vi "PNG Read.vi"(8 "error in (no error)":errorcluster, 11 "Image Path (*.png)":path) -> (0 "error out":errorcluster, 2 "Chunks":T1[](array[typedef]) {"CRC" format="%08x"}, 3 "dup Image Path":path)   [LabVIEW 2018, in "Export-Built-ins.lvlib"]
doc: "Returns the PNG image chunks from the <b>Image Path (*.png)</b>.\n\n<b>Errors:</b>\n1059: \"Unsupported file type\" if <b>Image Path (*.png)</b> is not a valid PNG file.\n\nCreated by: Ryan Pacini"
uses:
  Export-Built-ins.lvlib
  Controls/PNG Chunk.ctl
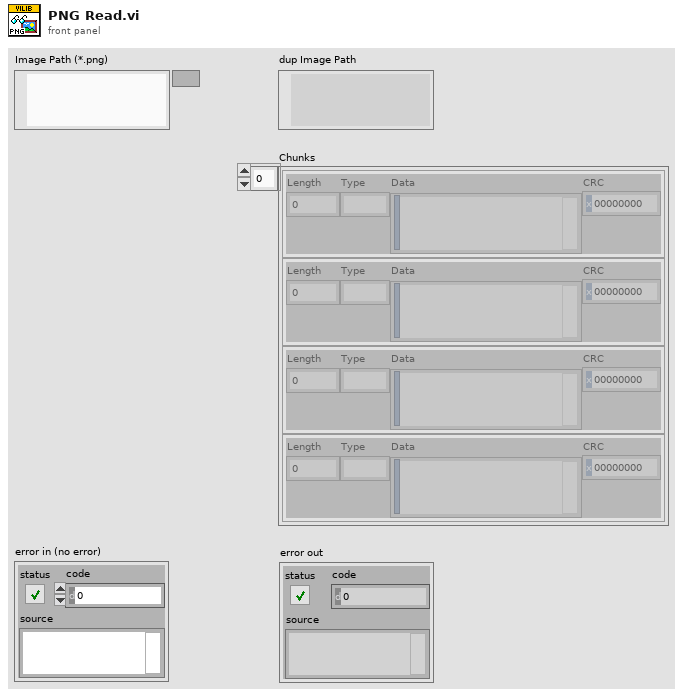
[diagram p1: front panel]
types:
  T1 = typedef "Export-Built-ins.lvlib/PNG Chunk.ctl" = cluster{"Length":i32, "Type":string, "Data":string, "CRC":u32}
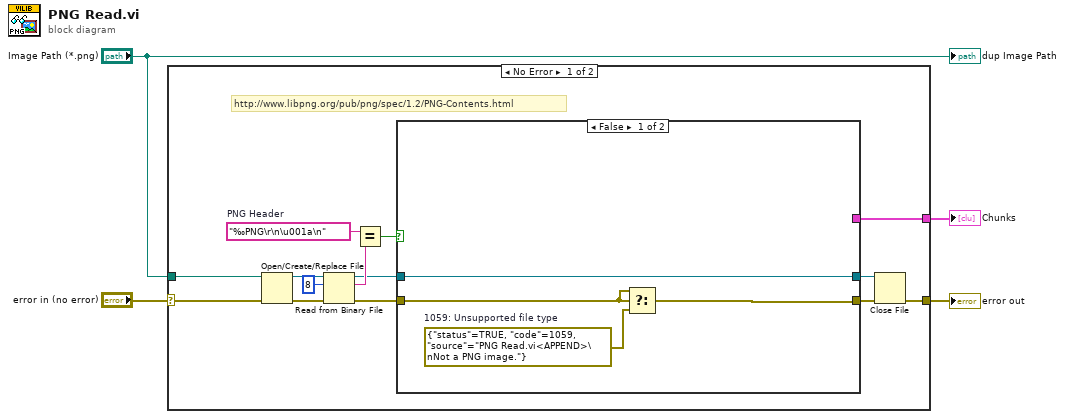
[diagram p0: block diagram]
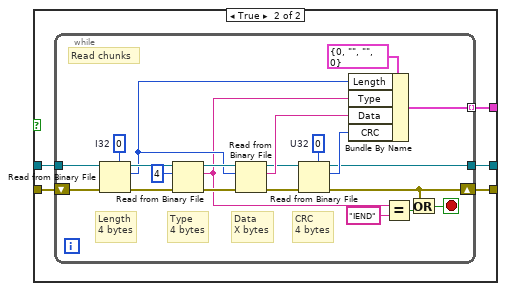
[diagram p2: hidden frame]
diagram:
  n1 = case shown="No Error" "error in (no error)" {
    selector: "error in (no error)" -> [w18 w50]
    tunnel: "Image Path (*.png)" -> [w17 _]
    tunnel: [w11 _] -> w2
    tunnel: [w9 w50] -> w3
    frame No Error {
      w5 = "‰PNG\r\n\u001a\n"  # PNG Header
      # "http://www.libpng.org/pub/png/spec/1.2/PNG-Contents.html"
      n2 = Open/Create/Replace File(file path (use dialog)=w17, error in=w18) -> (refnum out=w16:refnum<file>, error out=w15:errorcluster)  [unwired: 4 in, 1 out]
      n3 = Read from Binary File(8:w15, 10:8 ("count (1)"), 11:w16) -> (0:w13:errorcluster, 2:w14:string, 3:w12:refnum<file>)  [unwired: 3 in, 1 out]
      n4 = Equal?(x=w5, y=w14) -> (x = y?=w7:bool)
      n5 = case shown="False" w7 {
        tunnel: w13 -> [w21 w27]
        tunnel: w12 -> [w22 w26]
        tunnel: [_ w25] -> w11
        tunnel: [w20 w24] -> w10
        tunnel: [w22 w23] -> w8
        frame False {
          w19 = errorcluster {"status"=TRUE, "code"=1059, "source"="PNG Read.vi<APPEND>\nNot a PNG image."}  # 1059: Unsupported file type
          n6 = Select(t=w21, s=w21, f=w19) -> (s? t:f=w20:errorcluster)
        }
        frame True {
          n7 = while {
            tunnel: w26 -> [w48]
            tunnel: [w46] -> w25 mode=indexing
            shift-right: [w34] -> w24
            shift-left: w27 -> [w49]
            tunnel: [w30] -> w23
            stop <- w31 stop-if-true
            w36 = u32 0  # U32
            w47 = 0  # I32
            # "Read chunks"
            # "CRC\n4 bytes"
            # "Data\nX bytes"
            # "Type\n4 bytes"
            # "Length\n4 bytes"
            n8 = Read from Binary File(5:w47, 8:w49, 11:w48) -> (0:w45:errorcluster, 2:w40:i32, 3:w44:refnum<file>)  [unwired: 3 in, 1 out]
            n9 = Read from Binary File(8:w45, 10:4 ("count (1)"), 11:w44) -> (0:w42:errorcluster, 2:w33:string, 3:w41:refnum<file>)  [unwired: 3 in, 1 out]
            n10 = Read from Binary File(8:w42, 10:w40, 11:w41) -> (0:w38:errorcluster, 2:w39:string, 3:w37:refnum<file>)  [unwired: 3 in, 1 out]
            n11 = Read from Binary File(5:w36, 8:w38, 11:w37) -> (0:w34:errorcluster, 2:w35:u32, 3:w30:refnum<file>)  [unwired: 3 in, 1 out]
            n12 = Bundle By Name(cluster=T1 {"Length"=0, "Type"="", "Data"="", "CRC"=0} ("Chunk"), "Length"=w40, "Type"=w33, "Data"=w39, "CRC"=w35) -> (w46:T1)
            n13 = Equal?(x=w33, y="IEND") -> (x = y?=w32:bool)
            n14 = Or(x=w34, y=w32) -> (x .or. y?=w31:bool)
          }
        }
      }
      n15 = Close File(refnum=w8, error in=w10) -> (error out=w9:errorcluster)  [unwired: 1 out]
    }
    frame Error {
    }
  }
  "error out" <- w3
  "Chunks" <- w2
  "dup Image Path" <- "Image Path (*.png)"
